vi "Get_Registers.vi"(11 "Driver Filename":string) -> (3 "Registers":string[](array[string]))   [LabVIEW 2020, in "DriverCommon.lvlib"]
doc: "根据传输协议获得该协议支持的寄存器"
uses:
  DriverCommon.lvlib
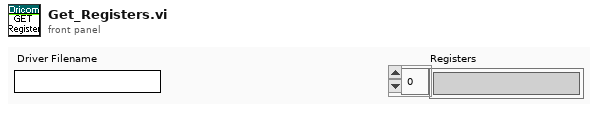
[diagram p1: front panel]
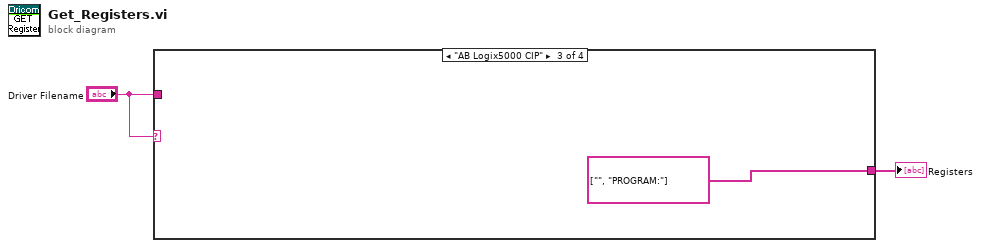
[diagram p0: block diagram]
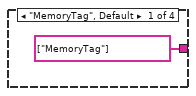
[diagram p2: hidden frame]
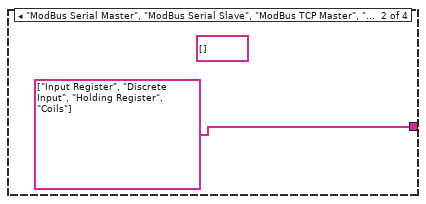
[diagram p3: hidden frame]
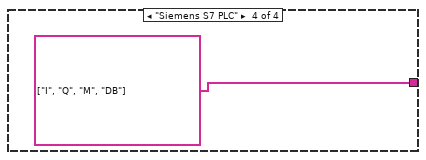
[diagram p4: hidden frame]
diagram:
  n1 = case shown="\"AB Logix5000 CIP\"" "Driver Filename" {
    tunnel: "Driver Filename" -> [_ _ _ _]
    tunnel: [string[] ["MemoryTag"] ("Registers") string[] ["Input Register", "Discrete Input", "Holding Register", "Coils"] ("Strings []") string[] ["", "PROGRAM:"] ("Registers") string[] ["I", "Q", "M", "DB"] ("Strings []")] -> w2
    frame "MemoryTag", Default {
    }
    frame "ModBus Serial Master", "ModBus Serial Slave", "ModBus TCP Master", "ModBus TCP Slave" {
      (unwired) string[] [] ("Registers")
    }
    frame "AB Logix5000 CIP" {
    }
    frame "Siemens S7 PLC" {
    }
  }
  "Registers" <- w2
